vi "tdsini.vi"(2 "Error In (No Error)":errorcluster, 3 "Acq_par":T1, 4 "VISA Port In":refnum<visa-resource-name>) -> (0 "Error Out":errorcluster, 1 "VISA Port Out":refnum<visa-resource-name>)   [LabVIEW 2011]
doc: "<B> Function </B> \nInitialize Oscilloscope. \nConfigure:\n- amount of averagings\n- number of sample points\n- sample rate"
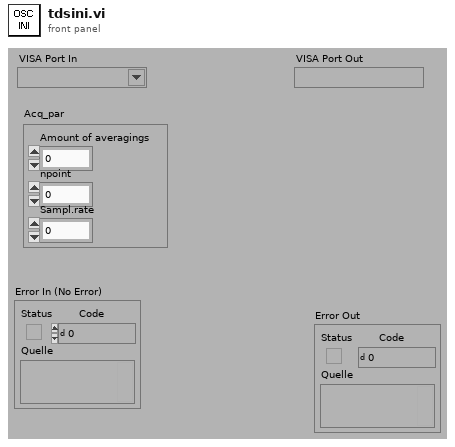
[diagram p1: front panel]
types:
  T1 = cluster{"Amount of averagings ":u32, "npoint":u32, "Sampl.rate":u64}
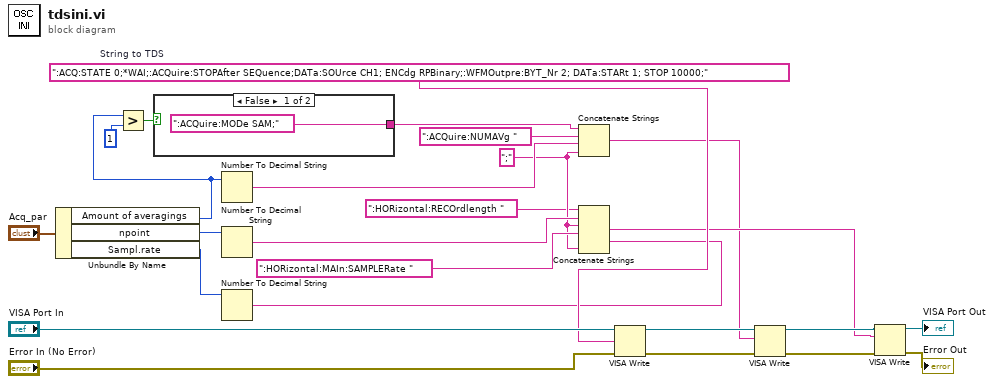
[diagram p0: block diagram]
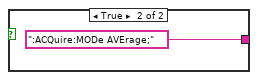
[diagram p2: hidden frame]
diagram:
  w8 = ";"
  w19 = ":ACQ:STATE 0;*WAI;:ACQuire:STOPAfter SEQuence;DATa:SOUrce CH1; ENCdg RPBinary;:WFMOutpre:BYT_Nr 2; DATa:STARt 1; STOP 10000;"  # String to TDS
  n1 = Unbundle By Name("Acq_par") -> ("Amount of averagings"=w4:u32, "npoint"=w17:u32, "Sampl.rate"=w16:u64)
  n2 = Greater?(x=w4, y=u32 1) -> (0:w2:bool)
  n3 = case shown="False" w2 {
    tunnel: [":ACQuire:MODe SAM;" ":ACQuire:MODe AVErage;"] -> w1
    frame False {
    }
    frame True {
    }
  }
  n4 = Number To Decimal String(number=w4) -> (decimal integer string=w22:string)  [unwired: 1 in]
  n5 = Number To Decimal String(number=w17) -> (decimal integer string=w11:string)  [unwired: 1 in]
  n6 = Number To Decimal String(number=w16) -> (decimal integer string=w9:string)  [unwired: 1 in]
  n7 = Concatenate Strings(w1, ":ACQuire:NUMAVg ", w22, w8) -> (w6:string)
  n8 = Concatenate Strings(":HORizontal:RECOrdlength ", w11, w8, ":HORizontal:MAIn:SAMPLERate ", w9, w8) -> (w7:string)
  n9 = VISA Write(VISA resource name="VISA Port In", write buffer=w19, error in (no error)="Error In (No Error)") -> (VISA resource name out=w15:refnum<visa-resource-name>, error out=w14:errorcluster)  [unwired: 1 out]
  n10 = VISA Write(VISA resource name=w15, write buffer=w6, error in (no error)=w14) -> (VISA resource name out=w13:refnum<visa-resource-name>, error out=w12:errorcluster)  [unwired: 1 out]
  n11 = VISA Write(VISA resource name=w13, write buffer=w7, error in (no error)=w12) -> (VISA resource name out=→"VISA Port Out":refnum<visa-resource-name>, error out=→"Error Out":errorcluster)  [unwired: 1 out]
